vi "AboutScreen.vi"(8 "error in (no error)":errorcluster) -> (0 "error out":errorcluster)   [LabVIEW 2018, in "ScreenGrabber.lvlib"]
uses:
  ScreenGrabber.lvlib
  <vilib>/event_ctls.llb/eventvkey.ctl
panel:
  # "Contacts:\nSivaramakrishnan, S <krishnansr.siva@gmail.com>\nSaishankar, N <sai.nshankar@gmail.com>"
  # "App Information:\n\nVersion: v1.2.1\nRelease Date: 19 January, 2019"
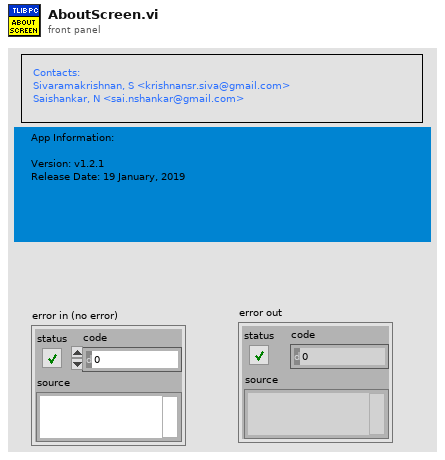
[diagram p1: front panel]
types:
  T1 = typedef "eventvkey.ctl" = enum16{"ASCII", "Enter", "Return", "Shift", "Ctrl", "Alt", "Cmd", "Opt", "Caps", "NumLock", "Clear", "Break", "Up", "Down", "Left", "Right", "Insert", "Delete", "Home", "End", "PageUp", "PageDown", "Escape", "Help", "Pause", "ScrollLock", "F1", "F2", "F3", "F4", "F5", "F6", "F7", "F8", "F9", "F10", "F11", "F12", "F13", "F14", "F15", "F16", "F17", "F18", "F19", "F20", "F21", "F22", "F23", "F24", "Play", "VolumeUp", "VolumeDown", "Mute", "Two Byte Char"}
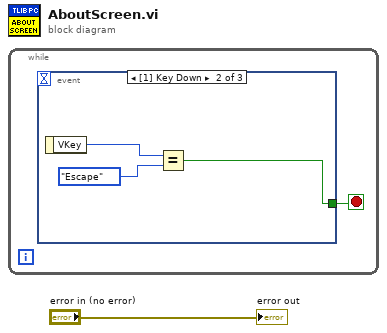
[diagram p0: block diagram]
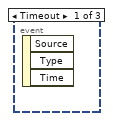
[diagram p2: hidden frame]
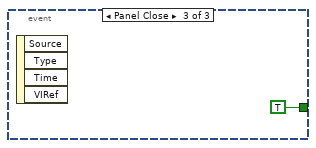
[diagram p3: hidden frame]
diagram:
  n1 = while {
    stop <- w2 stop-if-true
    n2 = event shown="[1] Key Down" {
      selector: _ -> [_ _ _]
      dyn-events: _ -> [_ _ _]
      timeout: _ -> [_ _ _]
      tunnel: [_ w3 TRUE] -> w2
      event Timeout {
        n3 = event-data() -> ()  [unwired: 1 in, 3 out]
      }
      event Key Down {
        n4 = event-data() -> ("VKey"=w5:T1)  [unwired: 1 in]
        n5 = Equal?(x=w5, y=eventvkey."Escape" ("VKey")) -> (x = y?=w3:bool)
      }
      event Panel Close {
        n6 = event-data() -> ()  [unwired: 1 in, 4 out]
      }
    }
  }
  "error out" <- "error in (no error)"
